vi "test Sensible Error If We Cancel A Future We Are Waiting On.vi"(8 "error in (no error)":errorcluster, 11 "TestCase in":refnum<class "Cancellation Tests.lvclass">) -> (0 "error out":errorcluster, 3 "TestCase out":refnum<class "Cancellation Tests.lvclass">)   [LabVIEW 2017, in "Cancellation Tests.lvclass"]
uses:
  Cancellation Tests.lvclass
  e9495466-0d5e-444b-a2d8-4487132dbe3c.vi
  <vilib>/addons/_JKI Toolkits/VI Tester/TestCase.llb/TestCase.lvclass
  Futures/Futures.lvlib
  Futures/Future/Future.lvclass
  C:/Program Files (x86)/National Instruments/LabVIEW 2017/vi.lib/addons/_JKI Toolkits/VI Tester/TestCase.llb/TestCase.lvclass
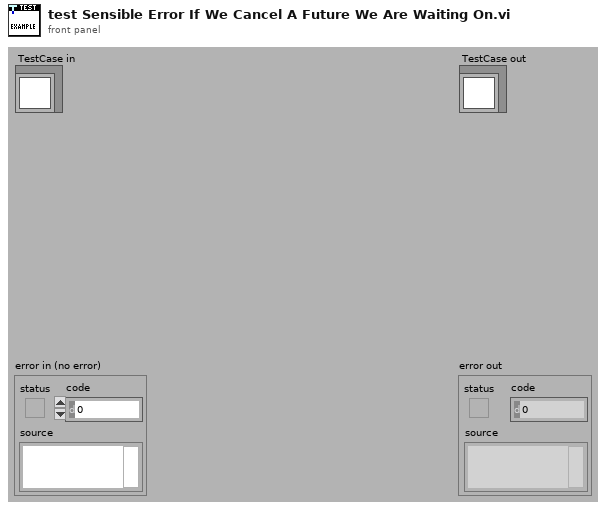
[diagram p1: front panel]
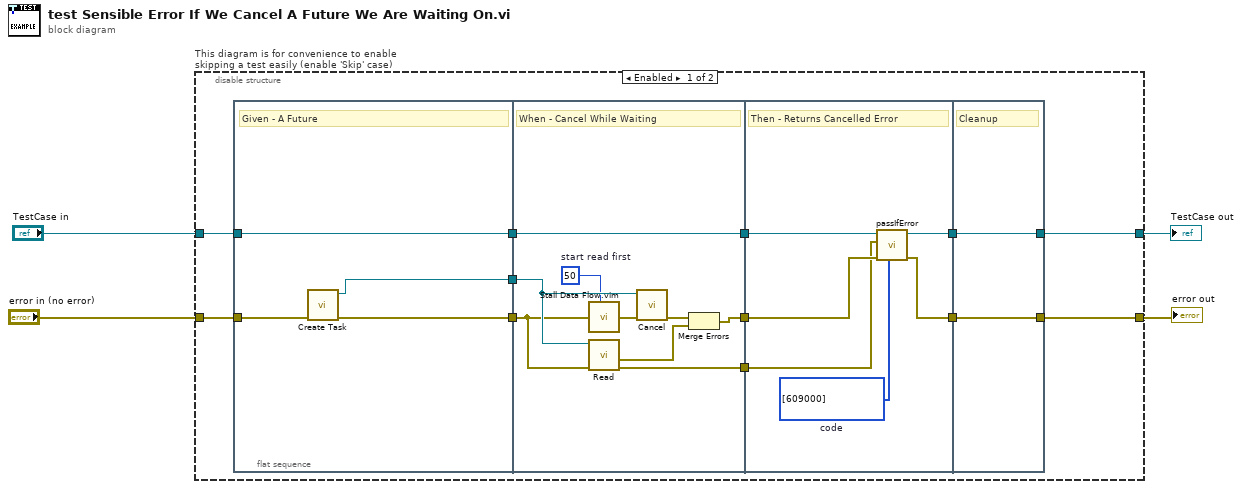
[diagram p0: block diagram]
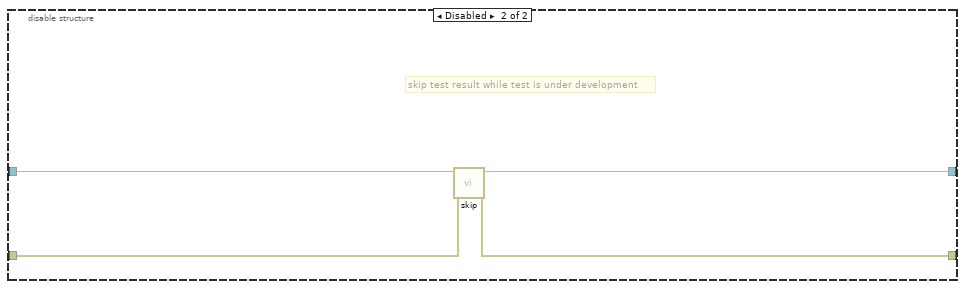
[diagram p2: hidden frame]
diagram:
  n1 = disable-structure "This diagram is for convenience to enable skipping a test easily (enable 'Skip' case)" shown="Enabled" {
    disable-tunnel: "TestCase in" -> [w12 w41]
    disable-tunnel: [w10 w39] -> w1
    disable-tunnel: [w9 w40] -> w3
    disable-tunnel: "error in (no error)" -> [w11 w38]
    frame Enabled {
      n2 = flat-sequence {
        tunnel: w11 -> [w19]
        tunnel: w12 -> [w20]
        tunnel: [w20] -> w16
        tunnel: [w18] -> w8
        tunnel: [w17] -> w7
        tunnel: [w29] -> w15
        tunnel: w16 -> [w29]
        tunnel: w8 -> [w24]
        tunnel: w7 -> [w27]
        tunnel: [w23] -> w6
        tunnel: [w21] -> w5
        tunnel: [w33] -> w14
        tunnel: [w35] -> w13
        tunnel: w15 -> [w34]
        tunnel: w6 -> [w32]
        tunnel: w5 -> [w31]
        tunnel: [w36] -> w9
        tunnel: [w37] -> w10
        tunnel: w14 -> [w37]
        tunnel: w13 -> [w36]
        frame #0 {
          # "Given - A Future"
          n3 = call "Create Task.vi"("error in (no error)"=w19) -> ("error out"=w18:errorcluster, "Future out"=w17:refnum<class "Future.lvclass">)  [unwired: 8 in, 1 out]
        }
        frame #1 {
          w25 = u32 50  # start read first
          # "When - Cancel While Waiting"
          n4 = call "Stall Data Flow.vim"("value in"=w24, "milliseconds to wait"=w25) -> ("value out"=w26:errorcluster)  [unwired: 1 out]
          n5 = call "Read.vi"("error in (no error)"=w24, "Future in"=w27) -> ("error out"=w21:errorcluster, "result error"=w22:errorcluster)  [unwired: 6 in, 2 out]
          n6 = call "Cancel.vi"("error in (no error)"=w26, "Future in"=w27) -> ("error out"=w28:errorcluster)  [unwired: 9 in]
          n7 = Merge Errors(w28, w22) -> (w23:errorcluster)
        }
        frame #2 {
          w30 = i32[] [609000]  # code
          # "Then - Returns Cancelled Error"
          n8 = call-dynamic "passIfError.vi"("passing error codes (default = any error code)"=w30, "error in (no error)"=w32, "error"=w31, "TestCase in"=w34) -> ("error out"=w35:errorcluster, "TestCase out"=w33:refnum<class "Cancellation Tests.lvclass">)  [unwired: 6 in]
        }
        frame #3 {
          # "Cleanup"
        }
      }
    }
    frame Disabled {
      # "skip test result while test is under development"
      n9 = call <vilib>:"skip.vi"("error in (no error)"=w38, "TestCase in"=w41) -> ("error out"=w40:errorcluster, "TestCase out"=w39:refnum<class "Cancellation Tests.lvclass">)  [unwired: 8 in]
    }
  }
  "error out" <- w3
  "TestCase out" <- w1
